vi "Table_Sort.vi"(9 "Sort Type":enum16{"numerical", "hex", "string"}(ring), 10 "Sort by":u16(ring) items=["Packet_Number", "Timestamp", "Source", "Destination", "Protocol", "Length", "Data"], 11 "Unsorted Data":string[][](array[string])=array1500x7[10500 elements]) -> (3 "Sorted data":string[][](array[string]))   [LabVIEW 2025, in "Automotive Ethernet Bus Monitor UI.lvlib" / "Table_Filtering.lvlib"]
uses:
  Table_Filtering.lvlib
  dd903b07-9a56-4d29-89d8-b4a603456dcb.vi
  <vilib>/Array/Sort 2D Array - Pop Stack.vi
  <vilib>/Array/Sort 2D Array - Push Stack.vi
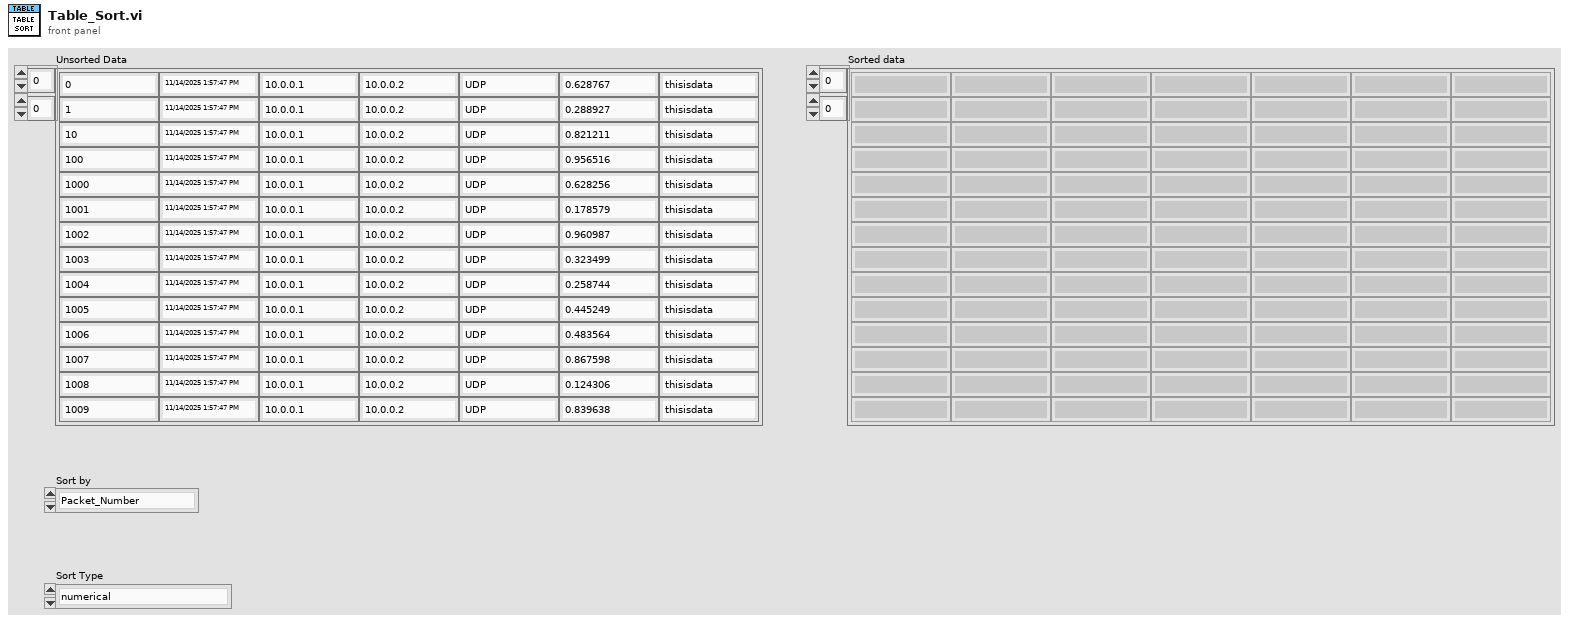
[diagram p1: front panel]
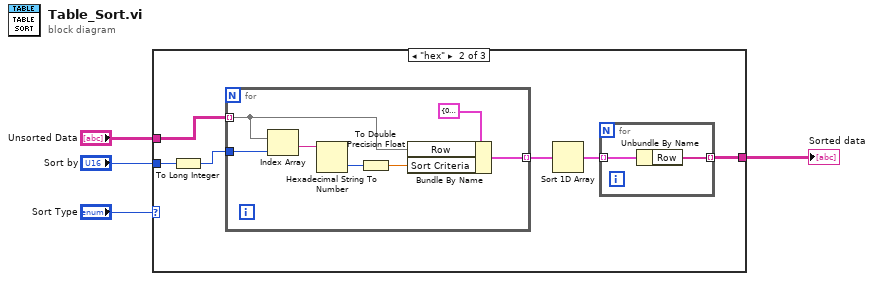
[diagram p0: block diagram]
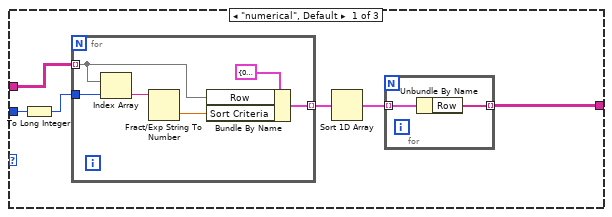
[diagram p2: hidden frame]
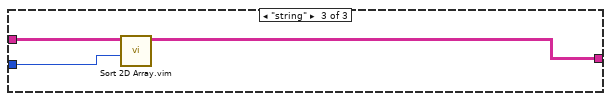
[diagram p3: hidden frame]
diagram:
  n1 = case shown="\"hex\"" "Sort Type" {
    tunnel: "Unsorted Data" -> [w10 w21 w36]
    tunnel: "Sort by" -> [w6 w19 w34]
    tunnel: [w7 w22 w35] -> w1
    frame "numerical", Default {
      n2 = To Long Integer(number=w6) -> (32bit integer=w5:i32)
      n3 = for {
        tunnel: w10 -> [w16] mode=indexing
        tunnel: [w14] -> w9 mode=indexing
        tunnel: w5 -> [w13]
        n4 = Index Array(array=w16, index=w13) -> (element=w18:string)
        n5 = Fract/Exp String To Number(string=w18) -> (number=w15:dbl)  [unwired: 3 in, 1 out]
        n6 = Bundle By Name(cluster=cluster{"Sort Criteria":dbl, "Row":string[]} {"Sort Criteria"=0.0, "Row"=[]}, "Row"=w16, "Sort Criteria"=w15) -> (w14:cluster{"Sort Criteria":dbl, "Row":string[]})
      }
      n7 = Sort 1D Array(array=w9) -> (sorted array=w8:cluster{"Sort Criteria":dbl, "Row":string[]}[])
      n8 = for {
        tunnel: w8 -> [w12] mode=indexing
        tunnel: [w11] -> w7 mode=indexing
        n9 = Unbundle By Name(w12) -> ("Row"=w11:string[])
      }
    }
    frame "hex" {
      n10 = To Long Integer(number=w19) -> (32bit integer=w20:i32)
      n11 = for {
        tunnel: w21 -> [w31] mode=indexing
        tunnel: w20 -> [w32]
        tunnel: [w30] -> w24 mode=indexing
        n12 = Index Array(array=w31, index=w32) -> (element=w29:string)
        n13 = Hexadecimal String To Number(string=w29) -> (number=w27:u32)  [unwired: 2 in, 1 out]
        n14 = To Double Precision Float(number=w27) -> (double precision float=w28:dbl)
        n15 = Bundle By Name(cluster=cluster{"Sort Criteria":dbl, "Row":string[]} {"Sort Criteria"=0.0, "Row"=[]}, "Row"=w31, "Sort Criteria"=w28) -> (w30:cluster{"Sort Criteria":dbl, "Row":string[]})
      }
      n16 = Sort 1D Array(array=w24) -> (sorted array=w23:cluster{"Sort Criteria":dbl, "Row":string[]}[])
      n17 = for {
        tunnel: w23 -> [w26] mode=indexing
        tunnel: [w25] -> w22 mode=indexing
        n18 = Unbundle By Name(w26) -> ("Row"=w25:string[])
      }
    }
    frame "string" {
      n19 = call "Sort 2D Array.vim"("index"=w34, "2D array"=w36) -> ("sorted 2D array"=w35:string[][])  [unwired: 8 in, 1 out]
    }
  }
  "Sorted data" <- w1
